vi "Dispose Buffer.vi"(8 "error in (no error)":errorcluster, 11 "Buffer in":refnum<class "Buffer.lvclass">) -> (0 "error out":errorcluster)   [LabVIEW 2017, in "DSF Core.lvlib" / "Buffer.lvclass"]
uses:
  Buffer.lvclass
  C:/Program Files (x86)/National Instruments/LabVIEW 2017/vi.lib/NI/Memory Manager/Classes/Pointer/Pointer.lvclass
  <vilib>/NI/Memory Manager/Classes/Pointer/Pointer.lvclass/Pointer.ctl
  <vilib>/NI/Memory Manager/Classes/Pointer/Protected/Parameter Checking/Check Null Pointer.vi
  <vilib>/NI/Memory Manager/Classes/Pointer/Private/Deallocate.vi
  <vilib>/NI/Memory Manager/Classes/Pointer/Protected/Errors.vi
  <vilib>/NI/Memory Manager/Classes/Pointer/Protected/Error VIs/Null Pointer.vi
  <vilib>/NI/Memory Manager/Classes/Pointer/API/Accessors/Get Address.vi
  <vilib>/NI/Memory Manager/Classes/Pointer/Protected/Get Internal.vi
  <vilib>/NI/Memory Manager/Classes/Pointer/Protected/Error VIs/Zone.vi
  <vilib>/NI/Memory Manager/Classes/Pointer/API/Accessors/Set Address.vi
  <vilib>/NI/Memory Manager/Classes/Pointer/API/Accessors/Set Size.vi
  <vilib>/NI/Memory Manager/Classes/Pointer/Private/Set Internal.vi
  <vilib>/NI/Memory Manager/Classes/Pointer/Protected/Error Building/Create Error.vi
  <vilib>/NI/Memory Manager/Constants/Constants.vi
  <vilib>/NI/Memory Manager/Constants/Library Name.vi
  <vilib>/NI/Memory Manager/Classes/Pointer/Protected/Error Building/Get Error Info.vi
  <vilib>/NI/Memory Manager/VIs/Write String into Source.vi
  <vilib>/NI/Memory Manager/VIs/Create Error Cluster.vi
  <vilib>/NI/Memory Manager/VIs/VIs for Poly/Create Error Cluster (256B).vi
  <vilib>/NI/Memory Manager/VIs/Set Error Status.vi
  <vilib>/NI/Memory Manager/VIs/Set Error Code.vi
  <vilib>/NI/Memory Manager/VIs/Set Error Source.vi
  <vilib>/NI/Memory Manager/Classes/Pointer/Pointer.lvclass
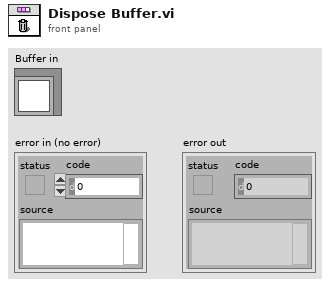
[diagram p1: front panel]
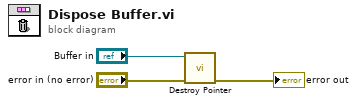
[diagram p0: block diagram]
diagram:
  n1 = call <vilib>:"Destroy Pointer.vi"("error in (no error)"="error in (no error)", "Pointer in"="Buffer in") -> ("error out"=→"error out":errorcluster)  [unwired: 8 in, 1 out]
